vi "Initialize.vi"(7 "Serial Configuration":T1={"Baud Rate"=57600, "Parity"=0, "Data Bits"=8, "Stop Bits"=10, "Flow Control"=0} {"Flow Control" items=["None", "XON/XOFF", "RTS/CTS", "XON/XOFF & RTS/CTS", "DTR/DSR", "XON/XOFF & DTR/DSR"]; "Stop Bits" items=["1.0"=10, "1.5"=15, "2.0"=20]; "Data Bits" items=["7"=7, "8"=8]; "Parity" items=["None", "Odd", "Even", "Mark", "Space"]; "Baud Rate" items=["300"=300, "600"=600, "1200"=1200, "2400"=2400, "4800"=4800, "9600"=9600, "19200"=19200, "38400"=38400, "57600"=57600, "115200"=115200]}, 8 "error in (no error)":errorcluster, 9 "Reset (True)":bool=TRUE, 10 "ID Query (True)":bool=TRUE, 11 "VISA resource name":refnum<visa-resource-name>) -> (0 "error out":errorcluster, 3 "VISA resource name out":refnum<visa-resource-name>)   [LabVIEW 2018, in "XP Power PLS600.lvlib"]
doc: "Establishes communication with the instrument and optionally performs an instrument identification query and/or an instrument reset. It also places the instrument in a default state needed for other instrument driver operations. Therefore, call this VI before calling other instrument driver VIs for this instrument. Generally, you need to call the Initialize VI only once at the beginning of an application."
uses:
  XP Power PLS600.lvlib
panel:
  # "(c) 2019 XP Power.  ALL RIGHTS RESERVED."
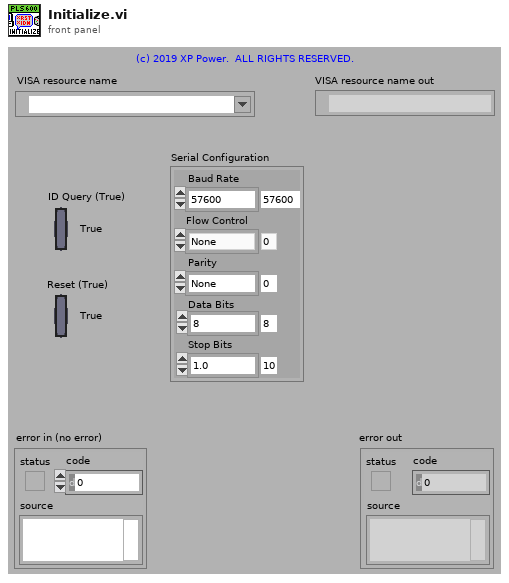
[diagram p1: front panel]
types:
  T1 = cluster{"Baud Rate":u32, "Parity":u16, "Data Bits":u16, "Stop Bits":u16, "Flow Control":u16}
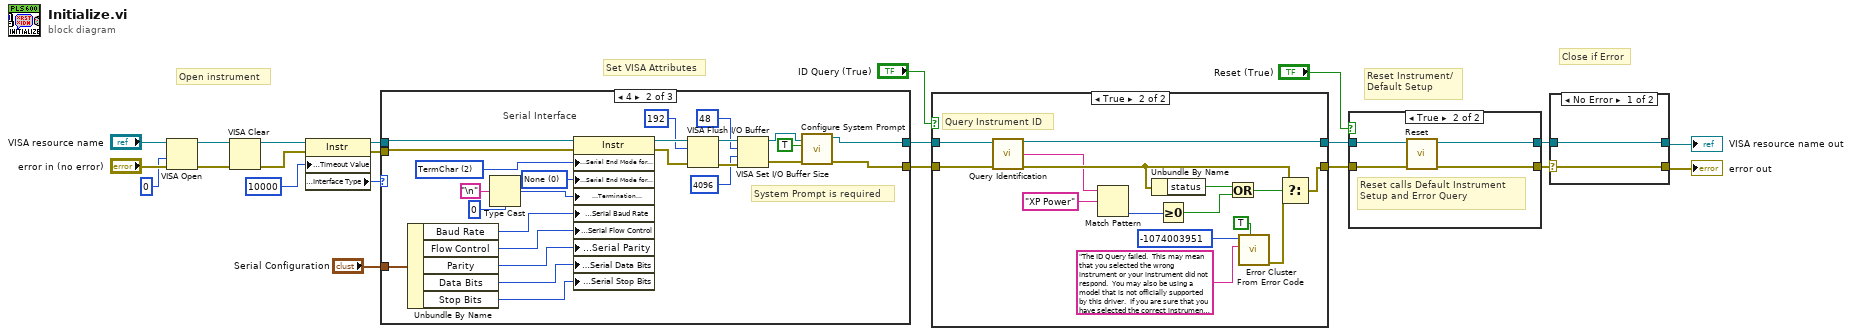
[diagram p0: block diagram]
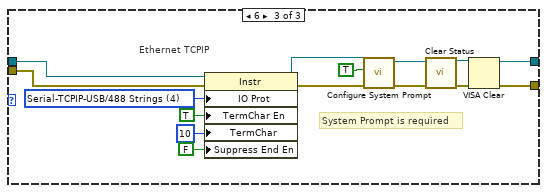
[diagram p3: hidden frame]
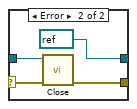
[diagram p4: hidden frame]
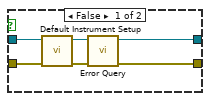
[diagram p5: hidden frame]
diagram:
  # "Set VISA Attributes"
  # "Close if Error"
  # "Reset Instrument/\nDefault Setup"
  # "Open instrument"
  n1 = VISA Open(access mode=u32 0, error in (no error)="error in (no error)", VISA resource name="VISA resource name") -> (VISA resource name=w10:refnum<visa-resource-name>, error out=w9:errorcluster)  [unwired: 2 in]
  n2 = VISA Clear(VISA resource name=w10, error in (no error)=w9) -> (VISA resource name out=w8:refnum<visa-resource-name>, error out=w7:errorcluster)
  n3 = property class="Instr"(reference=w8, error in=w7, "General Settings:Timeout Value"=u32 10000) -> (reference out=w13:refnum<visa-resource-name>, error out=w12:errorcluster, "Interface Information:Interface Type"=w1:u16)
  n4 = case shown="4" w1 {
    tunnel: [w23 w26 w60] -> w15
    tunnel: [w24 w25 w61] -> w14
    tunnel: w13 -> [w23 w48 w62]
    tunnel: w12 -> [w24 w49 w63]
    tunnel: "Serial Configuration" -> [_ w31 _]
    frame 0, Default {
      # "GPIB and USB Interface"
    }
    frame 4 {
      w30 = u16 0 items=["None", "Last Bit", "TermChar", "Break"] ("Serial Settings:End Mode for Writes")
      w38 = u16 2 items=["None", "LastBit", "TermChar"] ("Serial Settings:Serial End Mode for Reads")
      # "System Prompt is required"
      # "Serial Interface"
      n5 = Unbundle By Name(w31) -> ("Baud Rate"=w36:u32, "Flow Control"=w33:u16, "Parity"=w34:u16, "Data Bits"=w35:u16, "Stop Bits"=w32:u16)
      n6 = Type Cast(type=u8 0, x="\n" ("Line Feed Constant")) -> (*(type *) &x=w37:u8)
      n7 = property class="Instr"(reference=w48, error in=w49, "Serial Settings:Serial End Mode for Reads"=w38, "Serial Settings:Serial End Mode for Writes"=w30, "Message Based Settings:Termination Character"=w37, "Serial Settings:Serial Baud Rate"=w36, "Serial Settings:Serial Flow Control"=w33, "Serial Settings:Serial Parity"=w34, "Serial Settings:Serial Data Bits"=w35, "Serial Settings:Serial Stop Bits"=w32) -> (reference out=w44:refnum<visa-resource-name>, error out=w46:errorcluster)
      n8 = VISA Flush I/O Buffer(VISA resource name=w44, mask (16)=u16 192, error in (no error)=w46) -> (VISA resource name out=w47:refnum<visa-resource-name>, error out=w45:errorcluster)
      n9 = VISA Set I/O Buffer Size(VISA resource name=w47, mask (16)=u16 48, size (4096)=u32 4096 ("size (0)"), error in (no error)=w45) -> (VISA resource name out=w29:refnum<visa-resource-name>, error out=w28:errorcluster)
      n10 = call "Configure System Prompt.vi"("error in (no error)"=w28, "System Prompt State (F: Disable)"=TRUE, "VISA resource name"=w29) -> ("error out"=w25:errorcluster, "VISA resource name out"=w26:refnum<visa-resource-name>)  [unwired: 7 in]
    }
    frame 6 {
      w56 = u16 4 items=["Normal"=1, "VXI/FDC"=2, "GPIB/HS488"=3, "Serial-TCPIP-USB/488 Strings"=4, "USBTMC/Vendor-Specific"=5] ("Message Based Settings:IO Protocol")
      # "System Prompt is required"
      # "Ethernet TCPIP"
      n11 = property on="Property Node" class="Instr"(reference=w62, error in=w63, "IO Prot"=w56, "TermChar En"=TRUE ("Message Based Settings:Termination Character Enable"), "TermChar"=u8 10 ("Message Based Settings:Termination Character"), "Suppress End En"=FALSE ("Message Based Settings:Suppress End Enable")) -> (reference out=w52:refnum<visa-resource-name>, error out=w53:errorcluster)
      n12 = call "Configure System Prompt.vi"("error in (no error)"=w53, "System Prompt State (F: Disable)"=TRUE, "VISA resource name"=w52) -> ("error out"=w50:errorcluster, "VISA resource name out"=w51:refnum<visa-resource-name>)  [unwired: 7 in]
      n13 = call "Clear Status.vi"("VISA resource name"=w51, "error in (no error)"=w50) -> ("VISA resource name out"=w58:refnum<visa-resource-name>, "error out"=w59:errorcluster)  [unwired: 12 in]
      n14 = VISA Clear(VISA resource name=w58, error in (no error)=w59) -> (VISA resource name out=w60:refnum<visa-resource-name>, error out=w61:errorcluster)
    }
  }
  n15 = case shown="True" "ID Query (True)" {
    tunnel: [w65 w81] -> w21
    tunnel: [w66 w68] -> w22
    tunnel: w15 -> [w66 w67]
    tunnel: w14 -> [w65 w71]
    frame False {
    }
    frame True {
      # "Query Instrument ID"
      n16 = call "Query Identification.vi"("VISA resource name"=w67, "error in (no error)"=w71) -> ("VISA resource name out"=w68:refnum<visa-resource-name>, "Identification Response"=w69:string, "error out"=w70:errorcluster)  [unwired: 11 in]
      n17 = Match Pattern(string=w69, regular expression="XP Power") -> (offset past match=w75:i32)  [unwired: 1 in, 3 out]
      n18 = Unbundle By Name(w70) -> ("status"=w74:bool)
      n19 = Greater Or Equal To 0?(x=w75) -> (x >= 0?=w73:bool)
      n20 = Or(x=w74, y=w73) -> (x .or. y?=w72:bool)
      n21 = call <vilib>:"Error Cluster From Error Code.vi"("show call chain? (False)"=TRUE, "error message (\"\")"="The ID Query failed.  This may mean that you selected the wrong instrument or your instrument did not respond.  You may also be using a model that is not officially supported by this driver.  If you are sure that you have selected the correct instrument and it is responding, try disabling the ID Query." ("Source (VI Name)"), "error code (0)"=-1074003951 ("Code")) -> ("error out"=w79:errorcluster)  [unwired: 6 in]
      n22 = Select(t=w70, s=w72, f=w79) -> (s? t:f=w81:errorcluster)
    }
  }
  n23 = case shown="True" "Reset (True)" {
    tunnel: w21 -> [w86 w88]
    tunnel: [w84 w91] -> w3
    tunnel: w22 -> [w87 w89]
    tunnel: [w85 w90] -> w4
    frame False {
      n24 = call "Default Instrument Setup.vi"("error in (no error)"=w86, "VISA resource name"=w87) -> ("error out"=w82:errorcluster, "VISA resource name out"=w83:refnum<visa-resource-name>)  [unwired: 8 in]
      n25 = call "Error Query.vi"("error in (no error)"=w82, "VISA resource name"=w83) -> ("error out"=w84:errorcluster, "VISA resource name out"=w85:refnum<visa-resource-name>)  [unwired: 6 in, 2 out]
    }
    frame True {
      # "Reset calls Default Instrument Setup and Error Query"
      n26 = call "Reset.vi"("error in (no error)"=w88, "VISA resource name"=w89) -> ("error out"=w91:errorcluster, "VISA resource name out"=w90:refnum<visa-resource-name>)  [unwired: 8 in]
    }
  }
  n27 = case shown="No Error" w3 {
    selector: w3 -> [w92 w95]
    tunnel: w4 -> [w93 w96]
    tunnel: [w93 refnum<visa-resource-name> refnum ("VISA resource name out")] -> w6
    tunnel: [w92 w97] -> w5
    frame No Error {
    }
    frame Error {
      n28 = call "Close.vi"("error in (no error)"=w95, "VISA resource name"=w96) -> ("error out"=w97:errorcluster)  [unwired: 9 in]
    }
  }
  "VISA resource name out" <- w6
  "error out" <- w5
